vi "get DIM services.vi"(3 "can select all services":bool, 5 "error in (no error)":errorcluster) -> (15 "services":string[](array[string]), 17 "descriptors":string[](array[string]), 19 "error out":errorcluster)   [LabVIEW 2014, in "PTUtils.lvlib"]
uses:
  PTUtils.lvlib
  CSCore/CSSystem/CoreLib/CoreLib.lvlib
  CSlibraries/UtilityLib/UtilityLib.lvlib
  CSCore/CSSystem/CSSystemLib/CSSystemLib.lvlib
  CSlibraries-extern/DimLVEvent/LVDimInterface/LVDimInterface.lvlib
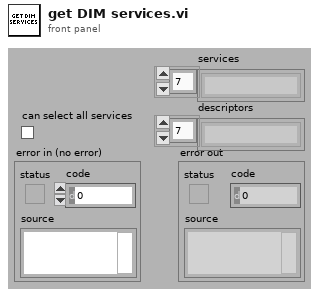
[diagram p1: front panel]
types:
  T1 = cluster{"string without white spaces":string, "string without white spaces":string}
  T2 = cluster{"string without white spaces":string, "string without white spaces":string}[]
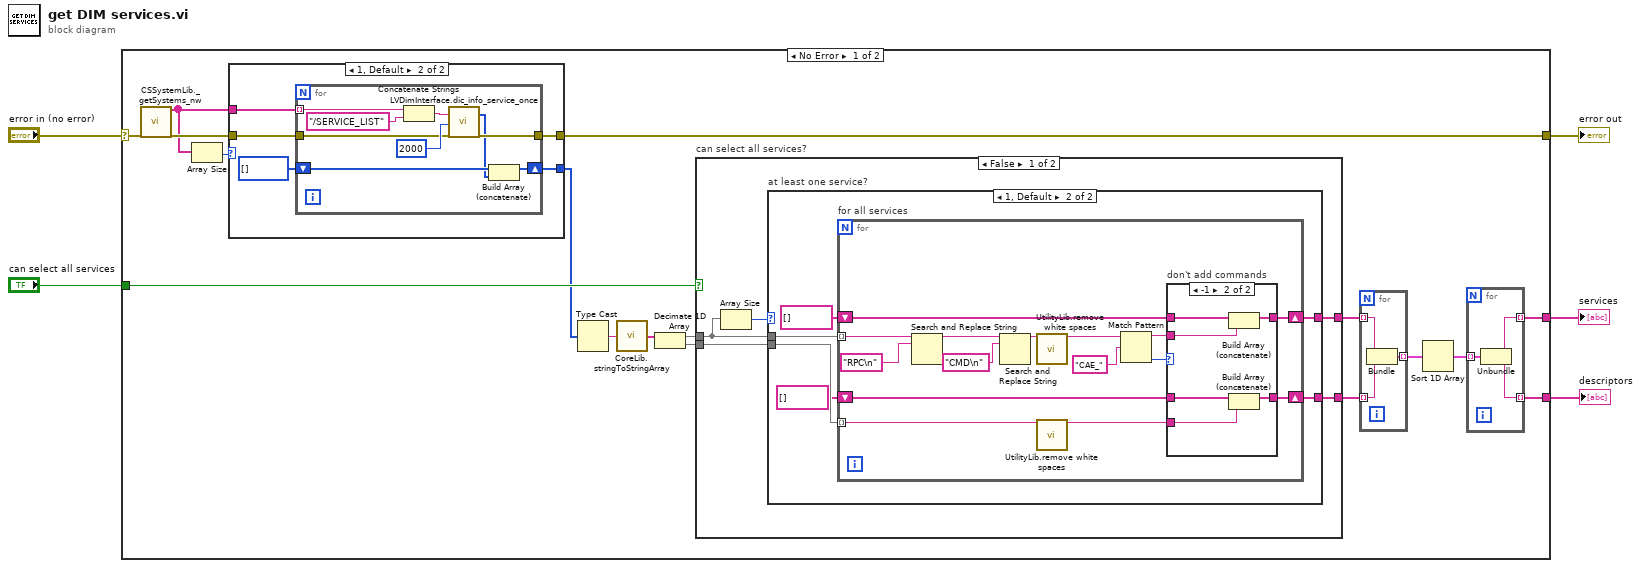
[diagram p0: block diagram]
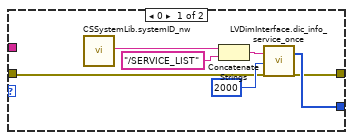
[diagram p2: hidden frame]
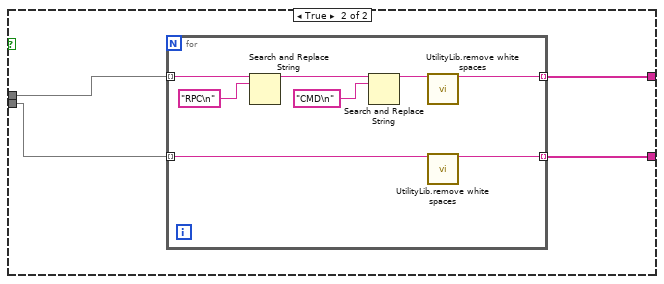
[diagram p5: hidden frame]
diagram:
  n1 = case shown="No Error" "error in (no error)" {
    selector: "error in (no error)" -> [w15 w96]
    tunnel: [w21 w96] -> w5
    tunnel: [w7 _] -> w4
    tunnel: "can select all services" -> [w22 _]
    tunnel: [w6 _] -> w1
    frame No Error {
      n2 = call "CSSystemLib._getSystems_nw.vi"("error in (no error)"=w15) -> ("CSSystems"=w14:string[], "error out"=w16:errorcluster)  [unwired: 16 in, 1 out]
      n3 = Array Size(array=w14) -> (size(s)=w13:i32)
      n4 = case shown="1, Default" w13 {
        tunnel: [w31 w40] -> w21
        tunnel: [w32 w39] -> w20
        tunnel: w16 -> [w30 w37]
        tunnel: w14 -> [_ w36]
        frame 0 {
          n5 = call "CSSystemLib.systemID_nw.vi"() -> ("systemID out"=w29:string)  [unwired: 18 in, 1 out]
          n6 = Concatenate Strings(w29, "/SERVICE_LIST" ("string")) -> (w34:string)
          n7 = call "LVDimInterface.dic_info_service_once.vi"("serviceName"=w34, "timeout [ms]"=u32 2000, "error in (no error)"=w30) -> ("data"=w32:i8[], "error out"=w31:errorcluster)  [unwired: 13 in, 2 out]
        }
        frame 1, Default {
          n8 = for {
            tunnel: [w49] -> w40
            shift-right: [w43] -> w39
            shift-left: i8[] [] ("data") -> [w45]
            tunnel: w36 -> [w46] mode=indexing
            tunnel: w37 -> [w42]
            n9 = Concatenate Strings(w46, "/SERVICE_LIST" ("string")) -> (w48:string)
            n10 = call "LVDimInterface.dic_info_service_once.vi"("serviceName"=w48, "timeout [ms]"=u32 2000, "error in (no error)"=w42) -> ("data"=w44:i8[], "error out"=w49:errorcluster)  [unwired: 13 in, 2 out]
            n11 = Build Array (concatenate)(w45, w44) -> (w43:i8[])
          }
        }
      }
      n12 = Type Cast(x=w20) -> (*(type *) &x=w17:string)  [unwired: 1 in]
      n13 = call "CoreLib.stringToStringArray.vi"("String"=w17) -> ("Array"=w19:string[])
      n14 = Decimate 1D Array(w19) -> (w18:string[], w12:string[])
      n15 = case "can select all services?" shown="False" w22 {
        tunnel: [w53 w86] -> w9
        tunnel: w18 -> [w52 w87]
        tunnel: w12 -> [w51 w84]
        tunnel: [w50 w85] -> w8
        frame False {
          n16 = Array Size(array=w52) -> (size(s)=w54:i32)
          n17 = case "at least one service?" shown="1, Default" w54 {
            tunnel: [_ w59] -> w53
            tunnel: w52 -> [_ w58]
            tunnel: w51 -> [_ w57]
            tunnel: [_ w55] -> w50
            frame 0 {
            }
            frame 1, Default {
              n18 = for "for all services" {
                shift-right: [w74] -> w59
                shift-left: string[] [] -> [w75]
                tunnel: w58 -> [w62] mode=indexing
                tunnel: w57 -> [w65] mode=indexing
                shift-right: [w66] -> w55
                shift-left: string[] [] -> [w67]
                n19 = Search and Replace String(input string=w62, search string="RPC\n" ("substring (\"\")")) -> (result string=w61:string)  [unwired: 6 in, 3 out]
                n20 = Search and Replace String(input string=w61, search string="CMD\n" ("substring (\"\")")) -> (result string=w72:string)  [unwired: 6 in, 3 out]
                n21 = call "UtilityLib.remove white spaces.vi"("string with blanks"=w72) -> ("string without white spaces"=w71:string)  [unwired: 14 in, 4 out]
                n22 = call "UtilityLib.remove white spaces.vi"("string with blanks"=w65) -> ("string without white spaces"=w64:string)  [unwired: 14 in, 4 out]
                n23 = Match Pattern(string=w71, regular expression="CAE_") -> (before substring=w68:string, offset past match=w69:i32)  [unwired: 1 in, 2 out]
                n24 = case "don't add commands" shown="-1" w69 {
                  tunnel: w75 -> [w77 w83]
                  tunnel: [w77 w82] -> w74
                  tunnel: w68 -> [_ w81]
                  tunnel: w67 -> [w76 w80]
                  tunnel: [w76 w79] -> w66
                  tunnel: w64 -> [_ w78]
                  frame 0, Default {
                  }
                  frame -1 {
                    n25 = Build Array (concatenate)(w83, w81) -> (w82:string[])
                    n26 = Build Array (concatenate)(w80, w78) -> (w79:string[])
                  }
                }
              }
            }
          }
        }
        frame True {
          n27 = for {
            tunnel: w87 -> [w89] mode=indexing
            tunnel: [w93] -> w86 mode=indexing
            tunnel: [w91] -> w85 mode=indexing
            tunnel: w84 -> [w92] mode=indexing
            n28 = Search and Replace String(input string=w89, search string="RPC\n" ("substring (\"\")")) -> (result string=w88:string)  [unwired: 6 in, 3 out]
            n29 = Search and Replace String(input string=w88, search string="CMD\n" ("substring (\"\")")) -> (result string=w94:string)  [unwired: 6 in, 3 out]
            n30 = call "UtilityLib.remove white spaces.vi"("string with blanks"=w94) -> ("string without white spaces"=w93:string)  [unwired: 14 in, 4 out]
            n31 = call "UtilityLib.remove white spaces.vi"("string with blanks"=w92) -> ("string without white spaces"=w91:string)  [unwired: 14 in, 4 out]
          }
        }
      }
      n32 = for {
        tunnel: w9 -> [w28] mode=indexing
        tunnel: w8 -> [w27] mode=indexing
        tunnel: [w26] -> w11 mode=indexing
        n33 = Bundle("string without white spaces"=w28, "string without white spaces"=w27) -> (w26:T1)  [unwired: 1 in]
      }
      n34 = Sort 1D Array(array=w11) -> (sorted array=w10:T2)
      n35 = for {
        tunnel: w10 -> [w25] mode=indexing
        tunnel: [w24] -> w7 mode=indexing
        tunnel: [w23] -> w6 mode=indexing
        n36 = Unbundle(w25) -> ("string without white spaces"=w24:string, "string without white spaces"=w23:string)
      }
    }
    frame Error {
    }
  }
  "error out" <- w5
  "services" <- w4
  "descriptors" <- w1
